vi "mod_Format Power Profile.vi"(1 "truncated burst":T1={"t0"=0.0, "dt"=1.0, "Y"=[]} {"Y" format="%.3f"; "dt" format="%^.2e"; "t0" format="%.4f"}, 2 "IQ Data":T1={"t0"=0.0, "dt"=1.0, "Y"=[]} {"Y" format="%.3f"; "dt" format="%^.2e"; "t0" format="%.4f"}) -> (0 "Power Profile":waveform(dbl)[](array[waveform]))   [LabVIEW 2020, in "niDMT.lvlib"]
uses:
  <vilib>/addons/Modulation/niDMT.lvlib
  <vilib>/addons/Modulation/Analog/controls/Complex Data Waveform.ctl
  <vilib>/addons/Modulation/niAMT.lvlib
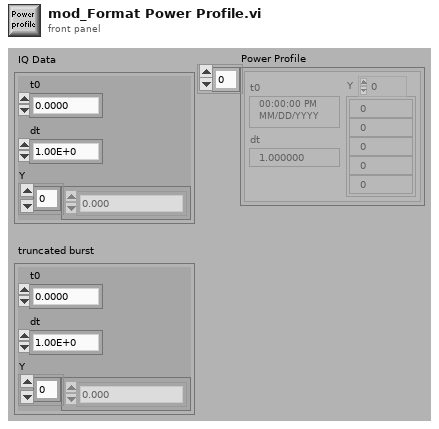
[diagram p1: front panel]
types:
  T1 = typedef "niAMT.lvlib/Complex Data Waveform.ctl" = cluster{"t0":dbl, "dt":dbl, "Y":cdb[]}
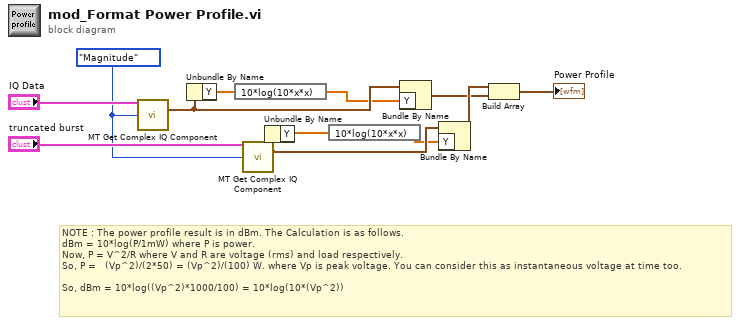
[diagram p0: block diagram]
diagram:
  w3 = enum16{"I", "Q", "Magnitude", "Phase"}."Magnitude" ("component choice")
  # "NOTE : The power profile result is in dBm. The Calculation is as follows.\ndBm = 10*log(P/1mW) where P is power. \nNow, P = V^2/R where V and R are voltage (rms) and load respectively. \nSo, P =   (Vp^2)/(2*50) = (Vp^2)/(100) W. where Vp is peak voltage. You can consider this as instantaneous voltage at time too. \n\nSo, dBm = 10*log((Vp^2)*1000/100) = 10*log(10*(Vp^2))"
  n1 = call <vilib>:"MT Get Complex IQ Component.vi"("IQ data (complex) in"="IQ Data", "component choice"=w3) -> ("CE component"=w7:waveform(dbl))  [unwired: 2 in, 11 out]
  n2 = Unbundle By Name(w7) -> ("Y"=w5:dbl[])
  n3 = expression code="10*log(10*x*x)"(w5) -> (w2:dbl[])
  n4 = call <vilib>:"MT Get Complex IQ Component.vi"("IQ data (complex) in"="truncated burst", "component choice"=w3) -> ("CE component"=w10:waveform(dbl))  [unwired: 2 in, 11 out]
  n5 = Unbundle By Name(w10) -> ("Y"=w8:dbl[])
  n6 = expression code="10*log(10*x*x)"(w8) -> (w1:dbl[])
  n7 = Bundle By Name(cluster=w7, "Y"=w2) -> (w9:waveform(dbl))
  n8 = Bundle By Name(cluster=w10, "Y"=w1) -> (w11:waveform(dbl))
  n9 = Build Array(w11, w9) -> (→"Power Profile":waveform(dbl)[])
